vi "(Depricated) Write Sample Push.Source Storage.vi"(10 "Sample Transfer Container":T1, 11 "cRIO-CO2 in":refnum<class "cRIO-CO2.lvclass">) -> (3 "cRIO-CO2 out":refnum<class "cRIO-CO2.lvclass">)   [LabVIEW 2015]
uses:
  cRIO-CO2.lvclass
  Controls/Sample Transfer Container Enumerator.ctl
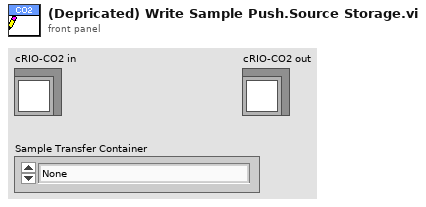
[diagram p1: front panel]
types:
  T1 = typedef "Sample Transfer Container Enumerator.ctl" = enum16{"None", "Sample 1", "Sample 2", "Sample 3", "Sample 4", "Sample 5", "Storage 01", "Storage 02", "Storage 03", "Storage 04", "Storage 05", "Storage 06", "Storage 07", "Storage 08", "Storage 09", "Storage 10", "Storage 11", "Storage 12", "Syringe", "Undefined"}
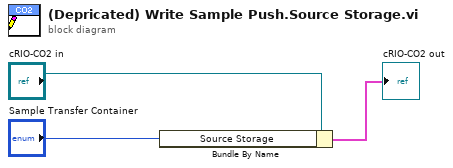
[diagram p0: block diagram]
diagram:
  n1 = Bundle By Name(cluster="cRIO-CO2 in", "Source Storage"="Sample Transfer Container") -> (→"cRIO-CO2 out":cluster{})
